vi "Stepper FPGA Rev B.vi"() -> ()   [LabVIEW 2014]
uses:
  <vilib>/rvi/Emulation/niFpgaGetClockAttributes.vi
  <vilib>/rvi/Emulation/niFpgaSctlEmulationGetInTimedLoop.vi
  <vilib>/rvi/Emulation/niFpgaEmulationReportErrorSimple.vi
  <vilib>/rvi/Emulation/niFpgaProcessEmulError.vi
  <vilib>/rvi/eio/common/nirviEmuTemplateMethod_errors.vi
  <vilib>/rvi/Emulation/niFpgaCriticalErrorInLSC.vi
  <vilib>/eio/EIONode/EIONode.xnode
panel:
  out "Steps to move":i32
  in  "Reset Step Counter":bool
  in  "Desired Position (Steps)":i32
  in  "Current (Steps)":i32
  in  "Step Period (uS)":i16
  in  "Enable/Disable Step Motor":bool
  out "Step Period":i16
  in  "Stop":bool
  out "Heartbeat":bool
  # "Motor Feedback"
  # "Motor Command"
  # "Choose a step period of 2000\nand a position of 400 to start"
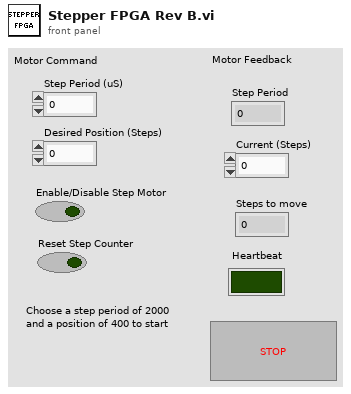
[diagram p1: front panel]
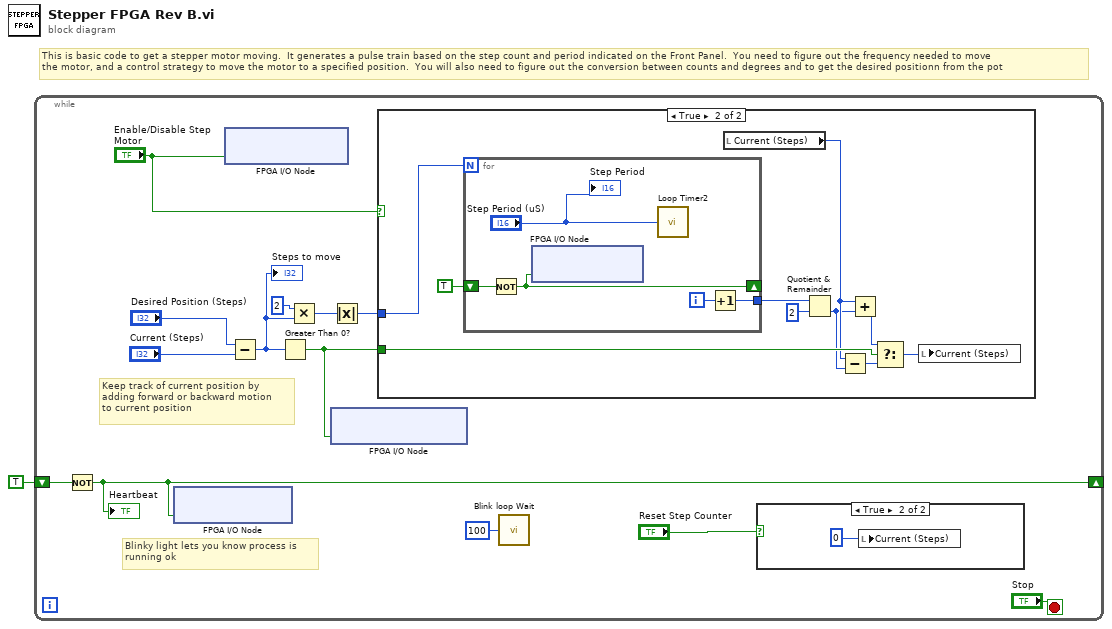
[diagram p0: block diagram]
diagram:
  # "This is basic code to get a stepper motor moving.  It generates a pulse train based on the step count and period indicated on the Front Panel.  You need to figure out the frequency needed to move \nthe motor, and a control strategy to move the motor to a specified position.  You will also need to figure out the conversion between counts and degrees and to get the desired positionn from the pot"
  n1 = while {
    shift-right: [w12] -> _
    shift-left: TRUE -> [w13]
    stop <- "Stop" stop-if-true
    # "Blinky light lets you know process is \nrunning ok"
    # "Keep track of current position by\nadding forward or backward motion\nto current position"
    n2 = Not(x=w13) -> (.not. x?=w12:bool)
    "Heartbeat" <- w12
    n3 = xnode "FPGA I/O Node"("Heartbeat LED"=w12) -> ()  [unwired: 1 in, 1 out]
    n4 = xnode "FPGA I/O Node"("Stepper_Enable"="Enable/Disable Step Motor") -> ()  [unwired: 1 in, 1 out]
    n5 = Subtract(x="Desired Position (Steps)", y="Current (Steps)") -> (x-y=w8:i32)
    "Steps to move" <- w8
    n6 = Greater Than 0?(x=w8) -> (x > 0?=w3:bool)
    n7 = Multiply(x=2, y=w8) -> (x*y=w7:i32)
    n8 = xnode "FPGA I/O Node"("Stepper_Direction"=w3) -> ()  [unwired: 1 in, 1 out]
    n9 = Absolute Value(x=w7) -> (abs(x)=w9:i32)
    n10 = case shown="True" "Enable/Disable Step Motor" {
      tunnel: w9 -> [_ w23]
      tunnel: w3 -> [_ w20]
      frame False {
      }
      frame True {
        n11 = for {
          N: w23 -> [_]
          shift-right: [w28] -> _
          shift-left: TRUE -> [w29]
          tunnel: [w25] -> w22
          i -> [w26]
          n12 = Not(x=w29) -> (.not. x?=w28:bool)
          n13 = xnode "FPGA I/O Node"("Stepper_Step"=w28) -> ()  [unwired: 1 in, 1 out]
          n14 = call "Loop Timer2"("Count(uSec)"="Step Period (uS)") -> ()  [unwired: 1 out]
          n15 = Increment(x=w26) -> (x+1=w25:i32)
          "Step Period" <- "Step Period (uS)"
        }
        n16 = local read "Current (Steps)"() -> (w17:i32)
        n17 = Quotient & Remainder(x=w22, y=2) -> (floor(x/y)=w16:i32)  [unwired: 1 out]
        n18 = Subtract(x=w17, y=w16) -> (x-y=w15:i32)
        n19 = Add(x=w17, y=w16) -> (x+y=w19:i32)
        n20 = Select(t=w19, s=w20, f=w15) -> (s? t:f=w18:i32)
        n21 = local write "Current (Steps)"(w18) -> ()
      }
    }
    n22 = call "Blink loop Wait"("Count(mSec)"=u32 100) -> ()  [unwired: 1 out]
    n23 = case shown="True" "Reset Step Counter" {
      frame False {
      }
      frame True {
        n24 = local write "Current (Steps)"(0 ("Current (Counts)")) -> ()
      }
    }
  }
